vi "Close Instrument Safely.vi"(8 "error in (no error)":errorcluster, 10 "Running (F)":bool, 11 "VISA Refnum in":refnum<visa-resource-name>) -> (0 "error out":errorcluster)   [LabVIEW 2020, in "ChromTech Series I Pump.lvlib" / "Instrument Manager.lvlib"]
doc: "Stops the pump if it is running, clears the character buffer on the pump, and closes the VISA resources given."
uses:
  process loops/Instrument Manager/Instrument Manager.lvlib
  <instrlib>/RxnRover/ChromtechSeriesIDriver/ChromTech Series I Drivers.lvlib
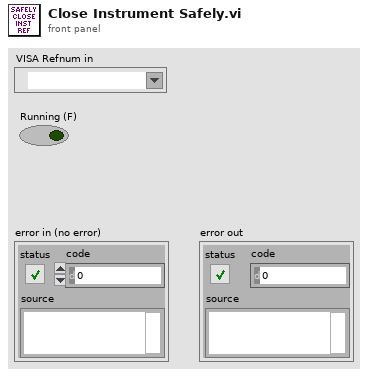
[diagram p1: front panel]
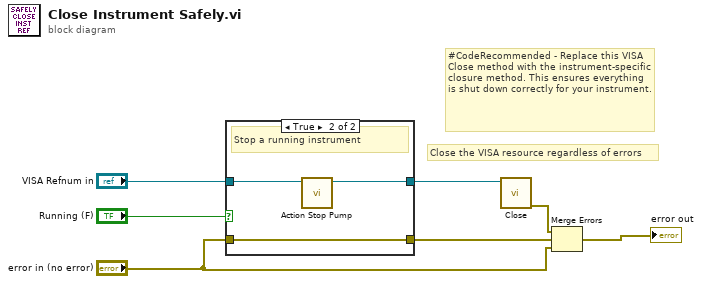
[diagram p0: block diagram]
diagram:
  # "#CodeRecommended - Replace this VISA Close method with the instrument-specific closure method. This ensures everything is shut down correctly for your instrument."
  # "Close the VISA resource regardless of errors"
  n1 = case shown="True" "Running (F)" {
    tunnel: "error in (no error)" -> [w9 w11]
    tunnel: [w9 w11] -> w2
    tunnel: "VISA Refnum in" -> [w8 w12]
    tunnel: [w8 w10] -> w5
    frame False {
    }
    frame True {
      # "Stop a running instrument"
      n2 = call <instrlib>:"Action Stop Pump.vi"("VISA resource name"=w12) -> ("VISA resource name out"=w10:refnum<visa-resource-name>)  [unwired: 9 in, 1 out]
    }
  }
  n3 = call <instrlib>:"Close.vi"("VISA resource name"=w5) -> ("error out"=w1:errorcluster)  [unwired: 10 in]
  n4 = Merge Errors(w1, w2, "error in (no error)") -> (→"error out":errorcluster)
